vi "FGVThreshold.vi"(7 "Enum":enum16{"write", "read"}(ring)=enum."read", 8 "error in (no error)":errorcluster, 11 "appended array 2":dbl[](array[numeric])) -> (0 "error in (no error) 2":errorcluster, 3 "appended array":dbl[](array[numeric]))   [LabVIEW 2022 SP3]
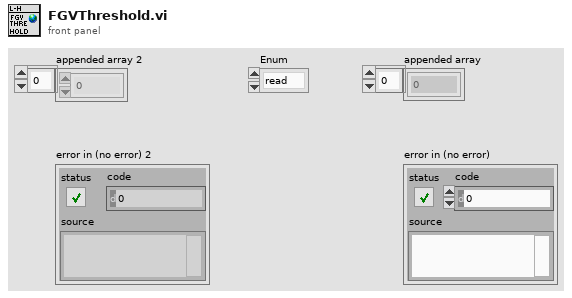
[diagram p1: front panel]
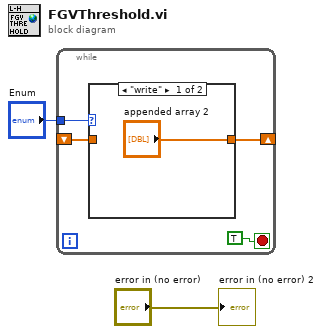
[diagram p0: block diagram]
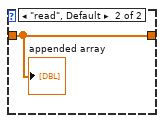
[diagram p2: hidden frame]
diagram:
  n1 = while {
    tunnel: "Enum" -> [w5]
    shift-right: [w4] -> _
    shift-left: _ -> [w3]
    stop <- TRUE stop-if-true
    n2 = case shown="\"write\"" w5 {
      tunnel: ["appended array 2" w8] -> w4
      tunnel: w3 -> [_ w8]
      frame "write" {
      }
      frame "read", Default {
        "appended array" <- w8
      }
    }
  }
  "error in (no error) 2" <- "error in (no error)"
